vi "Get_Data.vi"(8 "error in (no error)":errorcluster caption="entrée d'erreur (pas d'erreur)", 11 "Firebase Benches en entrée":refnum<class "Firebase AssembledProducts P1817.lvclass">) -> (0 "error out":errorcluster caption="sortie d'erreur", 3 "Firebase Benches en sortie":refnum<class "Firebase AssembledProducts P1817.lvclass">)   [LabVIEW 2020, in "Library Instrument & Equipement.lvlib" / "Library FireBase.lvlib" / "Firebase AssembledProducts P1817.lvclass"]
doc: "Returns all data Use Nb_To_Read to determine the number to read\nPlease initialise the following values\n - Name BDD\n - Document\n - API Key\n - Nb To Read"
uses:
  Firebase AssembledProducts P1817.lvclass
  C:/Users/ngarcin/OneDrive - Altyor/Standard TB/Class/Firebase/Source/Firebase Driver/Firebase Driver.lvclass
  Firebase AssembledProducts P1817.lvclass/Firebase AssembledProducts P1817.ctl
  JSON API/JSON Value/Set from JSON string.vi
  JSON API/JSON Value/JSON Value.lvclass
  Firebase Altyor/Firebase Altyor.lvclass
  JSON API/Variant JSON/Variant JSON.lvlib
  JSON API/Get Polymorphic/JSON GetSet.lvlib
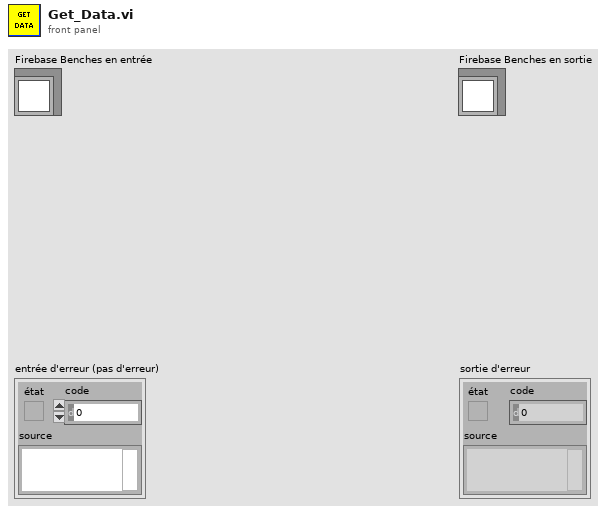
[diagram p1: front panel]
types:
  T1 = cluster{"name":string, "fields":cluster{"Result":cluster{"booleanValue":bool}, "CreationDate":cluster{"timestampValue":string}, "Batch":cluster{"stringValue":string}, "SerialNumber":cluster{"stringValue":string}, "EndOfProduction":cluster{"timestampValue":string}, "FW_Version":cluster{"mapValue":cluster{"fields":cluster{"Bootloader":cluster{"mapValue":cluster{"fields":cluster{"File_Name":cluster{"stringValue":string}, "Version":cluster{"mapValue":cluster{"fields":cluster{"Major":cluster{"stringValue":string}, "Minor":cluster{"stringValue":string}}}}, "Checksum":cluster{"stringValue":string}}}}, "SoftDevice":cluster{"mapValue":cluster{"fields":cluster{"File_Name":cluster{"stringValue":string}, "Version":cluster{"mapValue":cluster{"fields":cluster{"Major":cluster{"stringValue":string}, "Minor":cluster{"stringValue":string}}}}, "Checksum":cluster{"stringValue":string}}}}, "DFU":cluster{"mapValue":cluster{"fields":cluster{"File_Name":cluster{"stringValue":string}, "Version":cluster{"mapValue":cluster{"fields":cluster{"Major":cluster{"stringValue":string}, "Minor":cluster{"stringValue":string}}}}, "Checksum":cluster{"stringValue":string}}}}}}}, "PartNumber":cluster{"stringValue":string}, "OrderNumber":cluster{"stringValue":string}, "Operator":cluster{"stringValue":string}, "AssembledProductName":cluster{"stringValue":string}, "Delivery":cluster{"booleanValue":bool}}}[]
  T2 = cluster{"documents":cluster{"name":string, "fields":cluster{"Result":cluster{"booleanValue":bool}, "CreationDate":cluster{"timestampValue":string}, "Batch":cluster{"stringValue":string}, "SerialNumber":cluster{"stringValue":string}, "EndOfProduction":cluster{"timestampValue":string}, "FW_Version":cluster{"mapValue":cluster{"fields":cluster{"Bootloader":cluster{"mapValue":cluster{"fields":cluster{"File_Name":cluster{"stringValue":string}, "Version":cluster{"mapValue":cluster{"fields":cluster{"Major":cluster{"stringValue":string}, "Minor":cluster{"stringValue":string}}}}, "Checksum":cluster{"stringValue":string}}}}, "SoftDevice":cluster{"mapValue":cluster{"fields":cluster{"File_Name":cluster{"stringValue":string}, "Version":cluster{"mapValue":cluster{"fields":cluster{"Major":cluster{"stringValue":string}, "Minor":cluster{"stringValue":string}}}}, "Checksum":cluster{"stringValue":string}}}}, "DFU":cluster{"mapValue":cluster{"fields":cluster{"File_Name":cluster{"stringValue":string}, "Version":cluster{"mapValue":cluster{"fields":cluster{"Major":cluster{"stringValue":string}, "Minor":cluster{"stringValue":string}}}}, "Checksum":cluster{"stringValue":string}}}}}}}, "PartNumber":cluster{"stringValue":string}, "OrderNumber":cluster{"stringValue":string}, "Operator":cluster{"stringValue":string}, "AssembledProductName":cluster{"stringValue":string}, "Delivery":cluster{"booleanValue":bool}}}[], "nextPageToken":string}
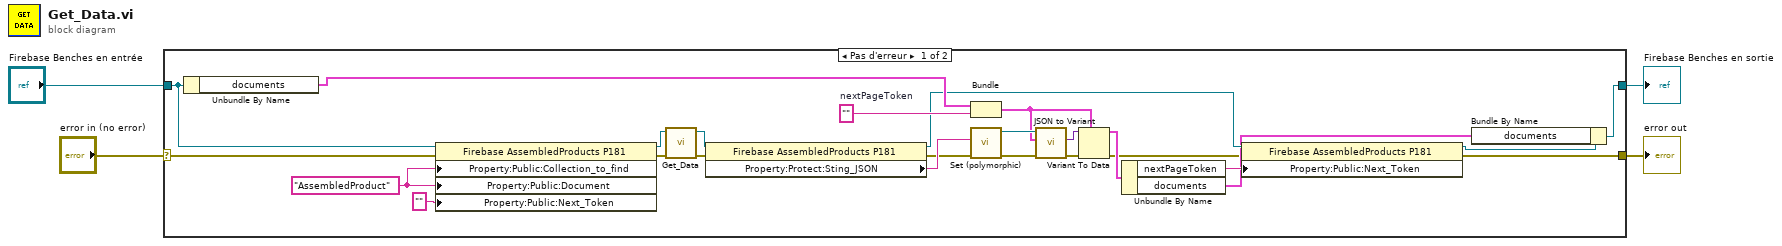
[diagram p0: block diagram]
diagram:
  n1 = case shown="Pas d'erreur" "error in (no error)" {
    selector: "error in (no error)" -> [w8 w31]
    tunnel: [w12 w30] -> w4
    tunnel: "Firebase Benches en entrée" -> [w7 w30]
    tunnel: [w9 w31] -> w2
    frame No Error {
      w6 = "AssembledProduct" ("Collection_to_find")
      w21 = ""  # nextPageToken
      n2 = Unbundle By Name(w7) -> ("documents"=w20:T1)
      n3 = property class="Firebase AssembledProducts P181"(reference=w7, error in=w8, "Property:Public:Collection_to_find"=w6, "Property:Public:Document"=w6, "Property:Public:Next_Token"="" ("Next_Token")) -> (reference out=w28:refnum<class "Firebase AssembledProducts P1817.lvclass">, error out=w27:errorcluster)
      n4 = call-parent "Get_Data.vi"("error in (no error)"=w27, "Firebase Altyor en entrée"=w28) -> ("error out"=w14:errorcluster, "Firebase Altyor en sortie"=w13:refnum<class "Firebase AssembledProducts P1817.lvclass">)  [unwired: 8 in]
      n5 = property class="Firebase AssembledProducts P181"(reference=w13, error in=w14) -> (reference out=w18:refnum<class "Firebase AssembledProducts P1817.lvclass">, error out=w11:errorcluster, "Property:Protect:Sting_JSON"=w23:string)
      n6 = Bundle("documents"=w20, "nextPageToken"=w21) -> (w19:T2)  [unwired: 1 in]
      n7 = call-poly "Set (polymorphic).vi"("error in (no error)"=w11, "JSON stream"=w23) -> ("error out"=w24:errorcluster, "JSON Value out"=w26:refnum<class "JSON Value.lvclass">)  [unwired: 7 in, 1 out]
      n8 = call "JSON to Variant.vi"("error in (no error)"=w24, "Variant (Data Type)"=w19, "JSON Value"=w26) -> ("error out"=w25:errorcluster, "Variant out"=w5:variant)  [unwired: 7 in]
      n9 = Variant To Data(error in=w25, type=w19, Variant=w5) -> (data=w22:T2, error out=w10:errorcluster)
      n10 = Unbundle By Name(w22) -> ("nextPageToken"=w17:string, "documents"=w15:T1)
      n11 = property class="Firebase AssembledProducts P181"(reference=w18, error in=w10, "Property:Public:Next_Token"=w17) -> (reference out=w16:refnum<class "Firebase AssembledProducts P1817.lvclass">, error out=w9:errorcluster)
      n12 = Bundle By Name(cluster=w16, "documents"=w15) -> (w12:refnum<class "Firebase AssembledProducts P1817.lvclass">)
    }
    frame Error {
    }
  }
  "Firebase Benches en sortie" <- w4
  "error out" <- w2
